vi "AK Befehl Auswerten_IAV Berlin.vi"(10 "Array":string[](array[string])) -> (2 "String für schreiben":string)   [LabVIEW 2020, in "AK-Schnittstelle.lvlib"]
uses:
  AK-Schnittstelle.lvlib
  Aktionen Stoernummern pruefen.ctl
  Aktionen Zustandsfehlerinformation.ctl
  AK Namen Aktionen.ctl
  Funktionstasten/Funktionstasten-Aktion.ctl
  Schedule Modul/Aktion FGV Scheduler Status.ctl
  Aktionen Gespeicherte Werte.ctl
  Seiten/FT-IR/FGV FT-IR Gasliste Aktionen.ctl
  Messdaten/Aktionen FGV Messdaten.ctl
  Funktionstasten/Zustaende.ctl
  Funktionstasten/Betriebsart.ctl
  Seiten/Log Konfig/Aktionen Trigger.ctl
  Funktionstasten/Funktionstasten.lvlib
  Seiten/Log Konfig/LogKonfig.lvlib
  Messdaten/Messdaten.lvlib
  Seiten/FT-IR/FT-IR.lvlib
  Schedule Modul/Schedule Modul.lvlib
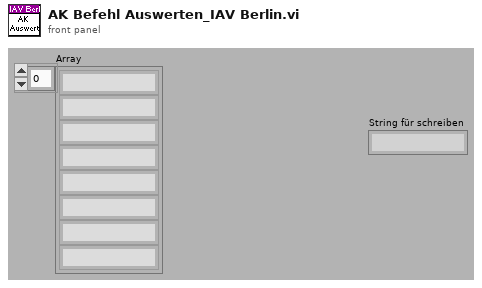
[diagram p1: front panel]
types:
  T1 = typedef "AK-Schnittstelle.lvlib/Aktionen Stoernummern pruefen.ctl" = enum16{"lesen", "prüfen"}
  T2 = typedef "AK-Schnittstelle.lvlib/Aktionen Zustandsfehlerinformation.ctl" = enum16{"OK", "Offline", "Busy", "Syntax Error", "Datenfehler"}
  T3 = typedef "AK-Schnittstelle.lvlib/AK Namen Aktionen.ctl" = enum16{"lesen", "laden", "speichern Namen", "AK Namen", "Liste erstellen", "EKFG erstellen", "speichern EKFG", "EKFG schreiben", "Neuen Eintrag erzeugen"}
  T4 = typedef "Schedule Modul.lvlib/Aktion FGV Scheduler Status.ctl" = enum16{"lesen", "init", "aktiv", "inaktiv"}
  T5 = typedef "Funktionstasten.lvlib/Funktionstasten-Aktion.ctl" = enum16{"Initialisieren", "Zustand setzen", "Taste gedrückt", "Fehler speichern", "Lesen", "Manuell", "Remote", "Bitparallel", "Samplepoint", "Zeit Prüfen", "reset Umschalten"}
  T6 = typedef "AK-Schnittstelle.lvlib/Aktionen Gespeicherte Werte.ctl" = enum16{"lesen", "laden", "speichern", "Seriell", "TCP", "Diverse", "AKTIV", "AK-Namen"}
  T7 = typedef "FT-IR.lvlib/FGV FT-IR Gasliste Aktionen.ctl" = enum16{"lesen", "Gasliste FT-IR", "Gasliste ausgelesen", "laden", "speichern", "löschen"}
  T8 = typedef "Messdaten.lvlib/Aktionen FGV Messdaten.ctl" = enum16{"lesen", "schreiben", "löschen", "Mittelwerte", "Komponente"}
  T9 = typedef "Funktionstasten.lvlib/Zustaende.ctl" = enum16{"Standby", "Pause", "Eco", "Messen", "Kalibrieren", "Spülen Filter", "Spülen Leitung", "Umgebungsluft", "0-Gas", "Cal-Gas", "CG zu PNS", "-------------", "Init 1", "Init 2", "Init 3", "Init 4", "Messen vorbereiten", "Messen durchführen", "Exit"}
  T10 = typedef "Funktionstasten.lvlib/Betriebsart.ctl" = enum16{"Manuell", "Remote", "Bitparallel"}
  T11 = typedef "LogKonfig.lvlib/Aktionen Trigger.ctl" = enum16{"lesen", "ALLE schreiben", "Trigger prüfen", "Trigger rücksetzen"}
  T12 = typedef "AK-Schnittstelle.lvlib/Diverse gespeicherte Werte.ctl" = cluster{"Kalibriergaseingang":i16, "SamplePoint":i16, "CalGas zu PNS":i16, "Gas-Reihenfolge":i16[], "Zeit 0-Gas":sgl, "Zeit CalGas":sgl, "AK Befehlssatz":T13}
  T13 = typedef "AK-Schnittstelle.lvlib/AK Befehlssatz.ctl" = enum16{"MEXA", "IAG v1.4", "AVL (Puma)", "PEUS"}
  T14 = typedef "String - Ausgabefeld.ctl" = string
  T15 = typedef "LogKonfig.lvlib/Element Triggerereignisse.ctl" = cluster{"Trigger verwenden":T16, "Messwert":u16, "kl./gr.":u16, "Wert":sgl, "Puffergröße":sgl}
  T16 = typedef "LogKonfig.lvlib/Auswahlfeld aktiviert-deaktiviert.ctl" = u16
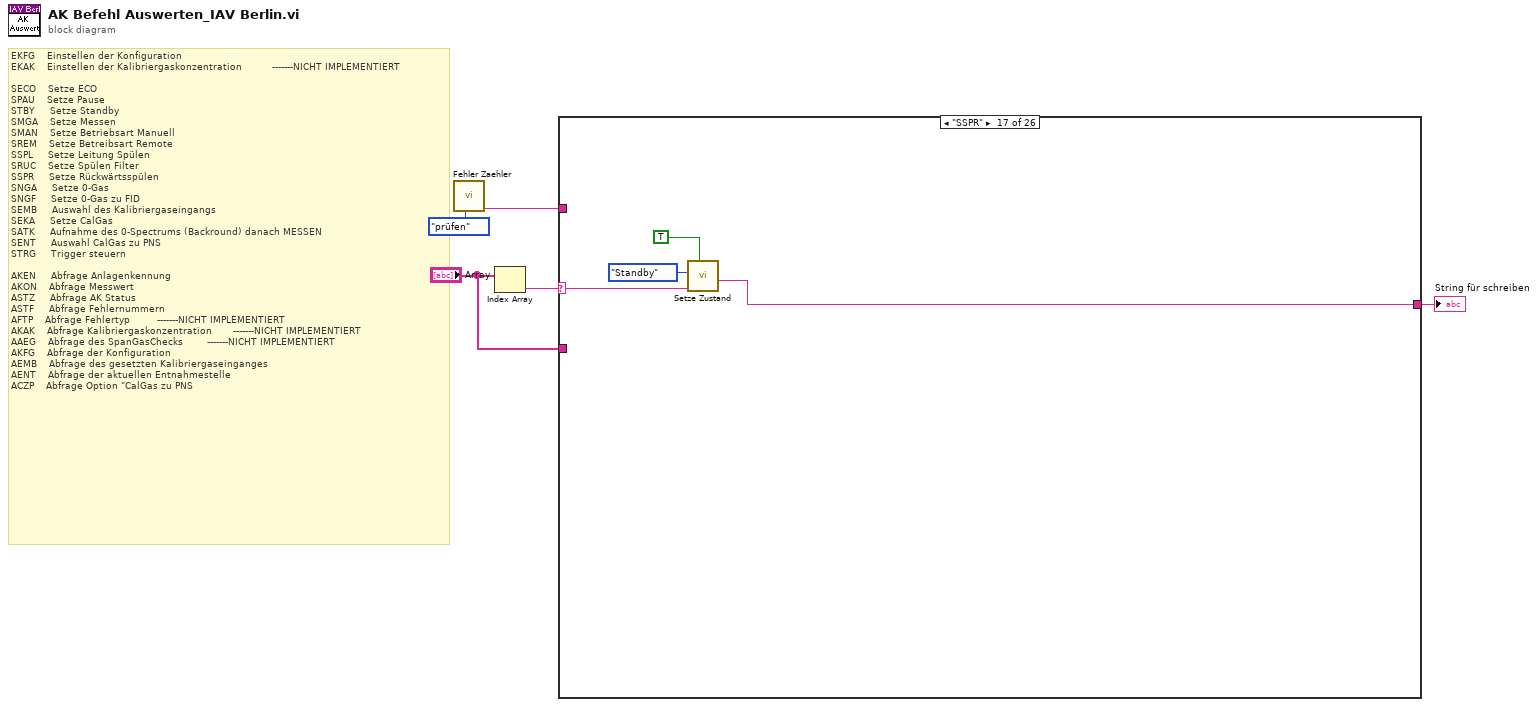
[diagram p0: block diagram]
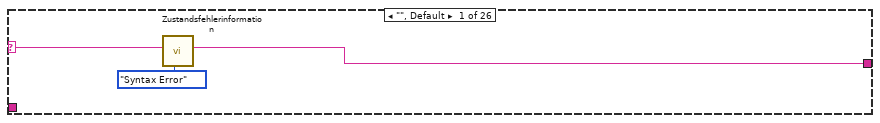
[diagram p2: hidden frame]
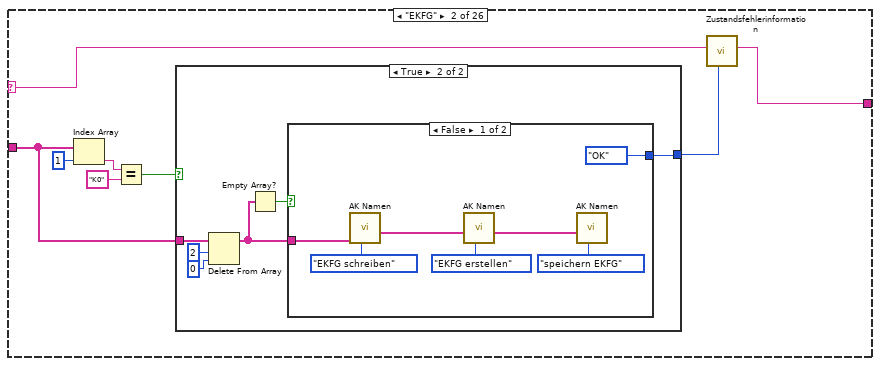
[diagram p3: hidden frame]
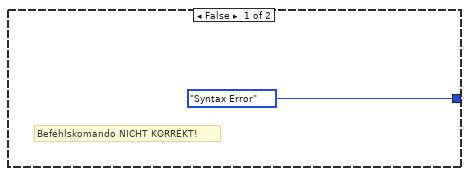
[diagram p4: hidden frame]
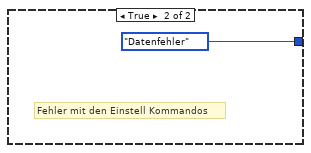
[diagram p5: hidden frame]
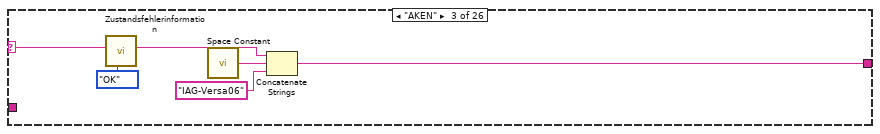
[diagram p6: hidden frame]
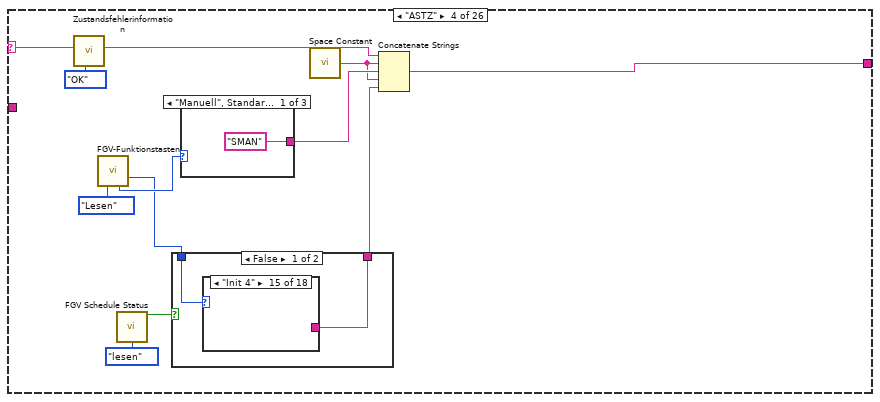
[diagram p7: hidden frame]
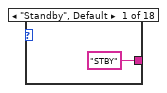
[diagram p8: hidden frame]
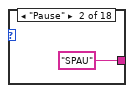
[diagram p9: hidden frame]
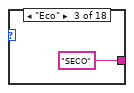
[diagram p10: hidden frame]
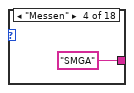
[diagram p11: hidden frame]
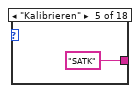
[diagram p12: hidden frame]
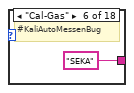
[diagram p13: hidden frame]
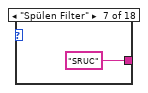
[diagram p14: hidden frame]
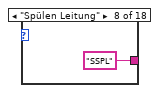
[diagram p15: hidden frame]
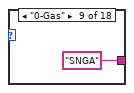
[diagram p16: hidden frame]
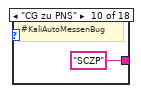
[diagram p17: hidden frame]
diagram:
  # "EKFG    Einstellen der Konfiguration\nEKAK    Einstellen der Kalibriergaskonzentration          -------NICHT IMPLEMENTIERT\n\nSECO    Setze ECO\nSPAU    Setze Pause\nSTBY     Setze Standby\nSMGA    Setze Messen\nSMAN    Setze Betriebsart Manuell\nSREM    Setze Betreibsart Remote\nSSPL     Setze Leitung Spülen\nSRUC    Setze Spülen Filter\nSSPR     Setze Rückwärtsspülen\nSNGA     Setze 0-Gas\nSNGF     Setze 0-Gas zu FID\nSEMB     Auswahl des Kalibriergaseingangs\nSEKA     Setze CalGas\nSATK     Aufnahme des 0-Spectrums (Backround) danach MESSEN\nSENT     Auswahl CalGas zu PNS\nSTRG     Trigger steuern\n\nAKEN     Abfrage Anlagenkennung\nAKON    Abfrage Messwert\nASTZ     Abfrage AK Status\nASTF     Abfrage Fehlernummern\nAFTP    Abfrage Fehlertyp         -------NICHT IMPLEMENTIERT\nAKAK    Abfrage Kalibriergaskonzentration       -------NICHT IMPLEMENTIERT\nAAEG    Abfrage des SpanGasChecks        -------NICHT IMPLEMENTIERT\nAKFG    Abfrage der Konfiguration\nAEMB    Abfrage des gesetzten Kalibriergaseinganges\nAENT    Abfrage der aktuellen Entnahmestelle\nACZP    Abfrage Option \"CalGas zu PNS"
  n1 = call "Fehler Zaehler.vi"("Aktionen"=Aktionen_Stoernummern_pruefen."prüfen") -> ("Fehlerzähler"=w3:string)  [unwired: 7 in, 3 out]
  n2 = Index Array(array="Array") -> (element=w2:string)  [unwired: 1 in]
  n3 = case shown="\"SSPR\"" w2 {
    selector: w2 -> [w7 w11 w34 w47 w70 w80 w89 w98 w109 w143 w189 w192 w195 w198 w201 w204 w208 w211 w215 w221 w230 w236 w260 w270 w278 w309]
    tunnel: [w6 w9 w36 w49 w72 w82 w91 w100 w111 w144 w188 w191 w194 w197 w200 w203 w207 w210 w214 w220 w229 w235 w259 w269 w277 w308] -> w5
    tunnel: w3 -> [_ _ _ _ _ _ _ _ _ _ _ _ _ _ _ _ _ _ _ _ _ _ _ _ _ _]
    tunnel: "Array" -> [_ w12 _ _ _ _ _ _ _ w134 _ _ _ _ _ _ _ _ _ _ _ w234 _ _ w276 w307]
    frame "", Default {
      n4 = call "Zustandsfehlerinformation.vi"("Aktionen"=Aktionen_Zustandsfehlerinformation."Syntax Error", "String"=w7) -> ("String"=w6:string)  [unwired: 9 in]
    }
    frame "EKFG" {
      n5 = Index Array(array=w12, index=1 ("Index")) -> (element=w15:string)
      n6 = Equal?(x=w15, y="K0") -> (x = y?=w13:bool)
      n7 = case shown="True" w13 {
        tunnel: w12 -> [_ w21]
        tunnel: [Aktionen_Zustandsfehlerinformation."Syntax Error" ("Aktionen") w18] -> w10
        frame False {
          # "Befehlskomando NICHT KORREKT!"
        }
        frame True {
          n8 = Delete From Array(array=w21, length=2 ("Länge"), index=0 ("Index")) -> (array with subset deleted=w20:string[])  [unwired: 1 out]
          n9 = Empty Array?(array=w20) -> (empty?=w19:bool)
          n10 = case shown="False" w19 {
            tunnel: w20 -> [w24 _]
            tunnel: [Aktionen_Zustandsfehlerinformation."OK" ("Aktionen") Aktionen_Zustandsfehlerinformation."Datenfehler" ("Aktionen")] -> w18
            frame False {
              n11 = call "AK Namen.vi"("Aktionen"=AK_Namen_Aktionen."EKFG schreiben", "EKFG Liste"=w24) -> ("AK Namen"=w27:string[])  [unwired: 6 in, 3 out]
              n12 = call "AK Namen.vi"("Aktionen"=AK_Namen_Aktionen."EKFG erstellen", "AK Namen"=w27) -> ("AK Namen"=w29:string[])  [unwired: 6 in, 3 out]
              n13 = call "AK Namen.vi"("Aktionen"=AK_Namen_Aktionen."speichern EKFG", "AK Namen"=w29) -> ()  [unwired: 6 in, 4 out]
            }
            frame True {
              # "Fehler mit den Einstell Kommandos"
            }
          }
        }
      }
      n14 = call "Zustandsfehlerinformation.vi"("Aktionen"=w10, "String"=w11) -> ("String"=w9:string)  [unwired: 9 in]
    }
    frame "AKEN" {
      n15 = call "Zustandsfehlerinformation.vi"("Aktionen"=Aktionen_Zustandsfehlerinformation."OK", "String"=w34) -> ("String"=w33:string)  [unwired: 9 in]
      n16 = call <vilib>:"Space Constant.vi"() -> ("String"=w32:string)
      n17 = Concatenate Strings(w33, w32, "IAG-Versa06" ("String")) -> (w36:string)
    }
    frame "ASTZ" {
      n18 = call "Zustandsfehlerinformation.vi"("Aktionen"=Aktionen_Zustandsfehlerinformation."OK", "String"=w47) -> ("String"=w46:string)  [unwired: 9 in]
      n19 = call "FGV-Funktionstasten.vi"("Aktion"=Funktionstasten-Aktion."Lesen") -> ("ausgewählte Funktion"=w39:T9, "Betriebsart"=w42:T10)  [unwired: 7 in, 6 out]
      n20 = call "FGV Schedule Status.vi"("Aktion"=Aktion_FGV_Scheduler_Status."lesen") -> ("Scheduler Status"=w40:bool)  [unwired: 13 in, 1 out]
      n21 = case shown="False" w40 {
        tunnel: w39 -> [w51 _]
        tunnel: [w50 "SATK" ("String")] -> w38
        frame False {
          n22 = case shown="\"Init 4\"" w51 {
            tunnel: ["STBY" ("String") "SPAU" ("String") "SECO" ("String") "SMGA" ("String") "SATK" ("String") "SEKA" ("String") "SRUC" ("String") "SSPL" ("String") "SNGA" ("String") "SCZP" ("String") _ _ _ _ _ _ _ _] -> w50
            frame "Standby", Default {
            }
            frame "Pause" {
            }
            frame "Eco" {
            }
            frame "Messen" {
            }
            frame "Kalibrieren" {
            }
            frame "Cal-Gas" {
              # "#KaliAutoMessenBug"
            }
            frame "Spülen Filter" {
            }
            frame "Spülen Leitung" {
            }
            frame "0-Gas" {
            }
            frame "CG zu PNS" {
              # "#KaliAutoMessenBug"
            }
            frame "Init 1" {
            }
            frame "Init 2" {
            }
            frame "-------------" {
            }
            frame "Init 3" {
            }
            frame "Init 4" {
            }
            frame "Messen vorbereiten" {
            }
            frame "Messen durchführen" {
            }
            frame "Exit" {
            }
          }
        }
        frame True {
        }
      }
      n23 = case shown="\"Manuell\", Standard" w42 {
        tunnel: ["SMAN" ("String") "SREM" ("String") "SBIT" ("String")] -> w44
        frame "Manuell", Default {
        }
        frame "Remote" {
        }
        frame "Bitparallel" {
        }
      }
      n24 = call <vilib>:"Space Constant.vi"() -> ("String"=w43:string)
      n25 = Concatenate Strings(w46, w43, w44, w43, w38) -> (w49:string)
    }
    frame "ASTF" {
      n26 = call "Zustandsfehlerinformation.vi"("Aktionen"=Aktionen_Zustandsfehlerinformation."OK", "String"=w70) -> ("String"=w69:string)  [unwired: 9 in]
      n27 = call "Fehler Zaehler.vi"("Aktionen"=Aktionen_Stoernummern_pruefen."lesen") -> ("Fehler Nummern"=w67:string)  [unwired: 7 in, 3 out]
      n28 = call <vilib>:"Space Constant.vi"() -> ("String"=w66:string)
      n29 = Concatenate Strings(w69, w66, w67) -> (w72:string)
    }
    frame "AEMB" {
      n30 = call "Zustandsfehlerinformation.vi"("Aktionen"=Aktionen_Zustandsfehlerinformation."OK", "String"=w80) -> ("String"=w79:string)  [unwired: 9 in]
      n31 = call "Gespeicherte Werte.vi"("Aktionen"=Aktionen_Gespeicherte_Werte."lesen") -> ("Diverse Werte"=w73:T12)  [unwired: 6 in, 4 out]
      n32 = Unbundle By Name(w73) -> ("Kalibriergaseingang"=w77:i16)
      n33 = call <vilib>:"Space Constant.vi"() -> ("String"=w74:string)
      n34 = Number To Decimal String(number=w77) -> (decimal integer string=w75:string)  [unwired: 1 in]
      n35 = Concatenate Strings(w79, w74, "M" ("String"), w75) -> (w82:string)
    }
    frame "AENT" {
      n36 = call "Zustandsfehlerinformation.vi"("Aktionen"=Aktionen_Zustandsfehlerinformation."OK", "String"=w89) -> ("String"=w88:string)  [unwired: 9 in]
      n37 = call "FGV-Funktionstasten.vi"("Aktion"=Funktionstasten-Aktion."Lesen") -> ("Samplepoint"=w83:u16)  [unwired: 7 in, 7 out]
      n38 = call <vilib>:"Space Constant.vi"() -> ("String"=w85:string)
      n39 = Number To Decimal String(number=w83) -> (decimal integer string=w86:string)  [unwired: 1 in]
      n40 = Concatenate Strings(w88, w85, "M" ("String"), w86) -> (w91:string)
    }
    frame "ACZP" {
      n41 = call "Zustandsfehlerinformation.vi"("Aktionen"=Aktionen_Zustandsfehlerinformation."OK", "String"=w98) -> ("String"=w97:string)  [unwired: 9 in]
      n42 = call "Gespeicherte Werte.vi"("Aktionen"=Aktionen_Gespeicherte_Werte."lesen") -> ("Diverse Werte"=w92:T12)  [unwired: 6 in, 4 out]
      n43 = Unbundle By Name(w92) -> ("CalGas zu PNS"=w95:i16)
      n44 = call <vilib>:"Space Constant.vi"() -> ("String"=w93:string)
      n45 = Number To Decimal String(number=w95) -> (decimal integer string=w94:string)  [unwired: 1 in]
      n46 = Concatenate Strings(w97, w93, w94) -> (w100:string)
    }
    frame "AKFG" {
      n47 = call "Gespeicherte Werte.vi"("Aktionen"=Aktionen_Gespeicherte_Werte."lesen") -> ("Diverse Werte"=w104:T12)  [unwired: 6 in, 4 out]
      n48 = Unbundle By Name(w104) -> ("Gas-Reihenfolge"=w106:i16[])
      n49 = call "FGV Gasliste.vi"("Aktionen"=FGV_FT-IR_Gasliste_Aktionen."lesen") -> ("Aktuelle Gasliste gesamt"=w101:T14[])  [unwired: 8 in, 2 out]
      n50 = for {
        tunnel: w106 -> [w120] mode=indexing
        shift-right: [w123] -> w103
        shift-left: "" -> [w122]
        tunnel: w101 -> [w121]
        i -> [w113]
        n51 = Index Array(array=w121, index=w120) -> (element=w118:T14)
        n52 = for {
          N: 10 -> [_]
          shift-right: [w128] -> w117
          shift-left: w118 -> [w129]
          stop <- w126 stop-if-true
          n53 = call <vilib>:"Space Constant.vi"() -> ("String"=w125:string)
          n54 = Search and Replace String(input string=w129, search string=w125, replace string="_") -> (result string=w128:string, number of replacements=w127:i32)  [unwired: 5 in, 2 out]
          n55 = Less Or Equal To 0?(x=w127) -> (x <= 0?=w126:bool)
        }
        n56 = Increment(x=w113) -> (x+1=w115:i32)
        n57 = Number To Decimal String(number=w115) -> (decimal integer string=w112:string)  [unwired: 1 in]
        n58 = call <vilib>:"Space Constant.vi"() -> ("String"=w116:string)
        n59 = Concatenate Strings(w122, w116, w117, w116, "K" ("String"), w112) -> (w123:string)
      }
      n60 = call "Zustandsfehlerinformation.vi"("Aktionen"=Aktionen_Zustandsfehlerinformation."OK", "String"=w109) -> ("String"=w108:string)  [unwired: 9 in]
      n61 = Concatenate Strings(w108, w103) -> (w111:string)
    }
    frame "AKON" {
      n62 = call "Gespeicherte Werte.vi"("Aktionen"=Aktionen_Gespeicherte_Werte."lesen") -> ("Diverse Werte"=w132:T12)  [unwired: 6 in, 4 out]
      n63 = Index Array(array=w134, index=1 ("Index")) -> (element=w137:string)
      n64 = Unbundle By Name(w132) -> ("Gas-Reihenfolge"=w140:i16[])
      n65 = Equal?(x=w137, y="K0") -> (x = y?=w135:bool)
      n66 = call "FGV Messdaten.vi"("Aktionen"=Aktionen_FGV_Messdaten."lesen") -> ("Aktuelle Messwerte"=w130:sgl[])  [unwired: 6 in, 8 out]
      n67 = case shown="False" w135 {
        tunnel: w140 -> [w147 w179]
        tunnel: [w145 w177] -> w139
        tunnel: w130 -> [w146 w176]
        tunnel: w134 -> [w151 _]
        tunnel: [w149 Aktionen_Zustandsfehlerinformation."OK" ("Aktionen")] -> w133
        frame False {
          n68 = Delete From Array(array=w151, length=1 ("Länge"), index=0 ("Index")) -> (array with subset deleted=w148:string[])  [unwired: 1 out]
          n69 = Empty Array?(array=w148) -> (empty?=w150:bool)
          n70 = case shown="False" w150 {
            tunnel: [Aktionen_Zustandsfehlerinformation."OK" ("Aktionen") Aktionen_Zustandsfehlerinformation."Datenfehler" ("Aktionen")] -> w149
            tunnel: w148 -> [w158 _]
            tunnel: w147 -> [w157 _]
            tunnel: w146 -> [w156 _]
            tunnel: [w155 ""] -> w145
            frame False {
              # "Je nach Abgefragten Kanal den RICHTIGEN\nMesswert heraussuchen!"
              n71 = for {
                tunnel: w158 -> [w172] mode=indexing
                tunnel: w157 -> [w170]
                tunnel: w156 -> [w169]
                shift-right: [w168] -> w155
                shift-left: "" -> [w165]
                n72 = Decimal String To Number(string=w172, offset=1 ("Offset (0)")) -> (number=w162:i32)  [unwired: 1 in, 1 out]
                n73 = Decrement(x=w162) -> (x-1=w161:i32)
                n74 = Index Array(array=w170, index=w161) -> (element=w164:i16)
                n75 = Decrement(x=w164) -> (x-1=w163:i16)
                n76 = Index Array(array=w169, index=w163) -> (element=w167:sgl)
                n77 = call <vilib>:"Space Constant.vi"() -> ("String"=w160:string)
                n78 = Number To Fractional String(number=w167) -> (F-format string=w166:string)  [unwired: 3 in]
                n79 = Concatenate Strings(w165, w160, w166) -> (w168:string)
              }
            }
            frame True {
              # "Wenn der String leer ist, dann Datenfehler"
            }
          }
        }
        frame True {
          n80 = for {
            tunnel: w179 -> [w180] mode=indexing
            shift-right: [w186] -> w177
            shift-left: "" -> [w185]
            tunnel: w176 -> [w184]
            n81 = Index Array(array=w184, index=w180) -> (element=w183:sgl)
            n82 = Number To Fractional String(number=w183) -> (F-format string=w182:string)  [unwired: 3 in]
            n83 = call <vilib>:"Space Constant.vi"() -> ("String"=w181:string)
            n84 = Concatenate Strings(w185, w181, w182) -> (w186:string)
          }
        }
      }
      n85 = call "Zustandsfehlerinformation.vi"("Aktionen"=w133, "String"=w143) -> ("String"=w142:string)  [unwired: 9 in]
      n86 = Concatenate Strings(w142, w139) -> (w144:string)
    }
    frame "SECO" {
      n87 = call "Setze Zustand.vi"("AK Befehl"=w189, "Zustand"=Zustaende."Eco") -> ("Antwort String"=w188:string)  [unwired: 8 in, 1 out]
    }
    frame "SPAU" {
      n88 = call "Setze Zustand.vi"("AK Befehl"=w192, "Zustand"=Zustaende."Pause") -> ("Antwort String"=w191:string)  [unwired: 8 in, 1 out]
    }
    frame "STBY" {
      n89 = call "Setze Zustand.vi"("AK Befehl"=w195, "Zustand"=Zustaende."Standby") -> ("Antwort String"=w194:string)  [unwired: 8 in, 1 out]
    }
    frame "SMGA" {
      n90 = call "Setze Zustand.vi"("AK Befehl"=w198, "Zustand"=Zustaende."Messen") -> ("Antwort String"=w197:string)  [unwired: 8 in, 1 out]
    }
    frame "SSPL" {
      n91 = call "Setze Zustand.vi"("AK Befehl"=w201, "Zustand"=Zustaende."Spülen Leitung") -> ("Antwort String"=w200:string)  [unwired: 8 in, 1 out]
    }
    frame "SRUC" {
      n92 = call "Setze Zustand.vi"("AK Befehl"=w204, "Zustand"=Zustaende."Spülen Filter") -> ("Antwort String"=w203:string)  [unwired: 8 in, 1 out]
    }
    frame "SSPR" {
      n93 = call "Setze Zustand.vi"("Befehl nicht vorhanden!"=TRUE, "AK Befehl"=w208, "Zustand"=Zustaende."Standby") -> ("Antwort String"=w207:string)  [unwired: 7 in, 1 out]
    }
    frame "SNGA" {
      n94 = call "Setze Zustand.vi"("AK Befehl"=w211, "Zustand"=Zustaende."0-Gas") -> ("Antwort String"=w210:string)  [unwired: 8 in, 1 out]
    }
    frame "SNGF" {
      n95 = call "Setze Zustand.vi"("Befehl nicht vorhanden!"=TRUE, "AK Befehl"=w215, "Zustand"=Zustaende."Standby") -> ("Antwort String"=w214:string)  [unwired: 7 in, 1 out]
    }
    frame "SMAN" {
      n96 = call "FGV-Funktionstasten.vi"("Aktion"=Funktionstasten-Aktion."Lesen") -> ("Betriebsart"=w217:T10)  [unwired: 7 in, 7 out]
      n97 = Equal?(x=Betriebsart."Remote" ("Betriebsart"), y=w217) -> (x = y?=w216:bool)
      n98 = case shown="True" w216 {
        tunnel: w221 -> [w224 w227]
        tunnel: [w222 w226] -> w220
        frame False {
          n99 = call "Zustandsfehlerinformation.vi"("Aktionen"=Aktionen_Zustandsfehlerinformation."Offline", "String"=w224) -> ("String"=w222:string)  [unwired: 9 in]
        }
        frame True {
          n100 = call "Zustandsfehlerinformation.vi"("Aktionen"=Aktionen_Zustandsfehlerinformation."OK", "String"=w227) -> ("String"=w226:string)  [unwired: 9 in]
          n101 = call "FGV-Funktionstasten.vi"("Aktion"=Funktionstasten-Aktion."Manuell") -> ()  [unwired: 7 in, 8 out]
        }
      }
    }
    frame "SREM" {
      n102 = call "Zustandsfehlerinformation.vi"("Aktionen"=Aktionen_Zustandsfehlerinformation."OK", "String"=w230) -> ("String"=w229:string)  [unwired: 9 in]
      n103 = call "FGV-Funktionstasten.vi"("Aktion"=Funktionstasten-Aktion."Remote") -> ()  [unwired: 7 in, 8 out]
    }
    frame "SEMB" {
      n104 = call "FGV-Funktionstasten.vi"("Aktion"=Funktionstasten-Aktion."Lesen") -> ("Betriebsart"=w233:T10)  [unwired: 7 in, 7 out]
      n105 = Equal?(x=Betriebsart."Remote" ("Betriebsart"), y=w233) -> (x = y?=w239:bool)
      n106 = case shown="True" w239 {
        tunnel: w236 -> [w241 w253]
        tunnel: [w240 w252] -> w235
        tunnel: w234 -> [_ w251]
        frame False {
          n107 = call "Zustandsfehlerinformation.vi"("Aktionen"=Aktionen_Zustandsfehlerinformation."Offline", "String"=w241) -> ("String"=w240:string)  [unwired: 9 in]
        }
        frame True {
          n108 = Index Array(array=w251, index=2 ("Index")) -> (element=w249:string)
          n109 = call "Zustandsfehlerinformation.vi"("Aktionen"=Aktionen_Zustandsfehlerinformation."OK", "String"=w253) -> ("String"=w252:string)  [unwired: 9 in]
          n110 = Decimal String To Number(string=w249, offset=1 ("Offset (0)")) -> (number=w245:i32)  [unwired: 1 in, 1 out]
          n111 = call "Gespeicherte Werte.vi"("Aktionen"=Aktionen_Gespeicherte_Werte."lesen") -> ("Diverse Werte"=w244:T12)  [unwired: 6 in, 4 out]
          n112 = Bundle By Name(cluster=w244, "Kalibriergaseingang"=w245) -> (w243:T12)
          n113 = call "Gespeicherte Werte.vi"("Aktionen"=Aktionen_Gespeicherte_Werte."Seriell", "Diverse Werte"=w243) -> ()  [unwired: 5 in, 5 out]
        }
      }
    }
    frame "SEKA" {
      n114 = call "FGV-Funktionstasten.vi"("Aktion"=Funktionstasten-Aktion."Lesen") -> ("Betriebsart"=w256:T10)  [unwired: 7 in, 7 out]
      n115 = Equal?(x=Betriebsart."Remote" ("Betriebsart"), y=w256) -> (x = y?=w255:bool)
      n116 = case shown="True" w255 {
        tunnel: w260 -> [w262 w267]
        tunnel: [w261 w266] -> w259
        frame False {
          n117 = call "Zustandsfehlerinformation.vi"("Aktionen"=Aktionen_Zustandsfehlerinformation."Offline", "String"=w262) -> ("String"=w261:string)  [unwired: 9 in]
        }
        frame True {
          n118 = call "Gespeicherte Werte.vi"("Aktionen"=Aktionen_Gespeicherte_Werte."lesen") -> ("Diverse Werte"=w264:T12)  [unwired: 6 in, 4 out]
          n119 = call "Zustandsfehlerinformation.vi"("Aktionen"=Aktionen_Zustandsfehlerinformation."OK", "String"=w267) -> ("String"=w266:string)  [unwired: 9 in]
          n120 = Unbundle By Name(w264) -> ()  [unwired: 1 out]
        }
      }
    }
    frame "SATK" {
      n121 = call "Setze Zustand.vi"("AK Befehl"=w270, "Zustand"=Zustaende."Kalibrieren") -> ("Antwort String"=w269:string)  [unwired: 8 in, 1 out]
    }
    frame "SENT" {
      n122 = call "FGV-Funktionstasten.vi"("Aktion"=Funktionstasten-Aktion."Lesen") -> ("Betriebsart"=w273:T10)  [unwired: 7 in, 7 out]
      n123 = Equal?(x=Betriebsart."Remote" ("Betriebsart"), y=w273) -> (x = y?=w272:bool)
      n124 = case shown="True" w272 {
        tunnel: w278 -> [w280 w296]
        tunnel: [w279 w295] -> w277
        tunnel: w276 -> [_ w294]
        frame False {
          n125 = call "Zustandsfehlerinformation.vi"("Aktionen"=Aktionen_Zustandsfehlerinformation."Offline", "String"=w280) -> ("String"=w279:string)  [unwired: 9 in]
        }
        frame True {
          n126 = Index Array(array=w294, index #1=2 ("Index"), index #2=3 ("Index")) -> (element #1=w292:string, element #2=w288:string)
          n127 = call "Zustandsfehlerinformation.vi"("Aktionen"=Aktionen_Zustandsfehlerinformation."OK", "String"=w296) -> ("String"=w295:string)  [unwired: 9 in]
          n128 = Empty String/Path?(string/path=w288) -> (empty?=w290:bool)
          n129 = case shown="True" w290 {
            tunnel: [w298 w301] -> w286
            tunnel: w288 -> [w299 _]
            frame False {
              n130 = Decimal String To Number(string=w299) -> (number=w298:i32)  [unwired: 2 in, 1 out]
            }
            frame True {
              n131 = call "Gespeicherte Werte.vi"("Aktionen"=Aktionen_Gespeicherte_Werte."lesen") -> ("Diverse Werte"=w300:T12)  [unwired: 6 in, 4 out]
              n132 = Unbundle By Name(w300) -> ("CalGas zu PNS"=w301:i16)
            }
          }
          n133 = Decimal String To Number(string=w292) -> (number=w282:i32)  [unwired: 2 in, 1 out]
          n134 = call "Gespeicherte Werte.vi"("Aktionen"=Aktionen_Gespeicherte_Werte."lesen") -> ("Diverse Werte"=w285:T12)  [unwired: 6 in, 4 out]
          n135 = Bundle By Name(cluster=w285, "SamplePoint"=w282, "CalGas zu PNS"=w286) -> (w284:T12)
          n136 = call "FGV-Funktionstasten.vi"("Samplepoint"=w282, "Aktion"=Funktionstasten-Aktion."Samplepoint") -> ()  [unwired: 6 in, 8 out]
          n137 = call "Gespeicherte Werte.vi"("Aktionen"=Aktionen_Gespeicherte_Werte."Seriell", "Diverse Werte"=w284) -> ()  [unwired: 5 in, 5 out]
        }
      }
    }
    frame "STRG" {
      n138 = call "FGV-Funktionstasten.vi"("Aktion"=Funktionstasten-Aktion."Lesen") -> ("Betriebsart"=w304:T10)  [unwired: 7 in, 7 out]
      n139 = Equal?(x=Betriebsart."Remote" ("Betriebsart"), y=w304) -> (x = y?=w303:bool)
      n140 = case shown="True" w303 {
        tunnel: w309 -> [w311 w318]
        tunnel: [w310 w317] -> w308
        tunnel: w307 -> [_ w316]
        frame False {
          n141 = call "Zustandsfehlerinformation.vi"("Aktionen"=Aktionen_Zustandsfehlerinformation."Offline", "String"=w311) -> ("String"=w310:string)  [unwired: 9 in]
        }
        frame True {
          n142 = Index Array(array=w316, index=2 ("Index")) -> (element=w314:string)
          n143 = call "Zustandsfehlerinformation.vi"("Aktionen"=Aktionen_Zustandsfehlerinformation."OK", "String"=w318) -> ("String"=w317:string)  [unwired: 9 in]
          n144 = Empty String/Path?(string/path=w314) -> (empty?=w313:bool)
          n145 = case shown="False" w313 {
            tunnel: w314 -> [w325 _]
            frame False {
              n146 = Decimal String To Number(string=w325) -> (number=w322:i32)  [unwired: 2 in, 1 out]
              n147 = call "FGV Trigger.vi"("Aktion"=Aktionen_Trigger."lesen") -> ("Triggerereignis neu"=w321:T15)  [unwired: 7 in, 3 out]
              n148 = Bundle By Name(cluster=w321, "Trigger verwenden"=w322) -> (w320:T15)
              n149 = call "FGV Trigger.vi"("Aktion"=Aktionen_Trigger."ALLE schreiben", "Triggerereignis"=w320) -> ()  [unwired: 6 in, 4 out]
            }
            frame True {
            }
          }
        }
      }
    }
  }
  "String für schreiben" <- w5
